vi "Distance.vi"() -> ()   [LabVIEW 2015]
panel:
  out "Distance":dbl
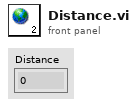
[diagram p1: front panel]
diagram:
